vi "CheckIfSubpanel.vi"(8 "error in":errorcluster, 11 "Subpanel Control Layout in":refnum<class "Subpanel Control Layout.lvclass">) -> (0 "error out":errorcluster, 2 "subpanel?":bool, 3 "Subpanel Control Layout out":refnum<class "Subpanel Control Layout.lvclass">)   [LabVIEW 2010, in "NI_SE_Front Panel Layout.lvlib" / "Subpanel Control Layout.lvclass"]
uses:
  Subpanel Control Layout.lvclass
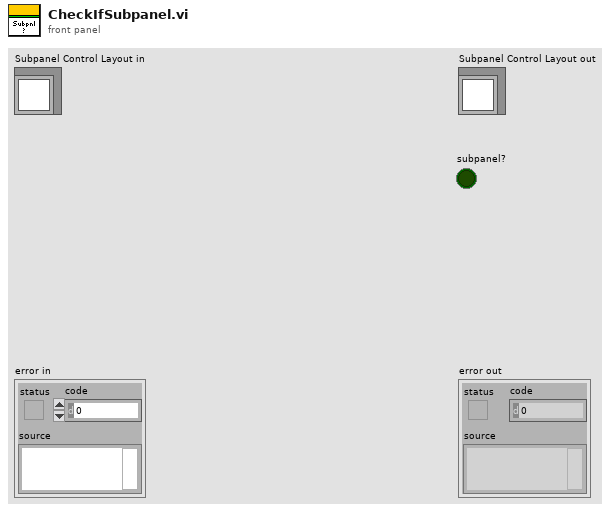
[diagram p1: front panel]
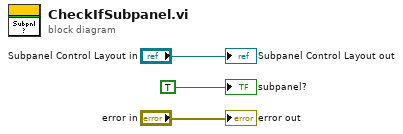
[diagram p0: block diagram]
diagram:
  "error out" <- "error in"
  "Subpanel Control Layout out" <- "Subpanel Control Layout in"
  "subpanel?" <- TRUE ("Boolean")
